vi "Timeout.vi"(11 "Squares type":T1[][](array[typedef])) -> (3 "Clicked Position":i32[](array[numeric]))   [LabVIEW 2019]
uses:
  #typedef_SquareType.ctl
  #typedef_Color.ctl
  #typedef_Piece.ctl
  #typedef_PieceType.ctl
panel:
  out "?":u16[][](array[ring])
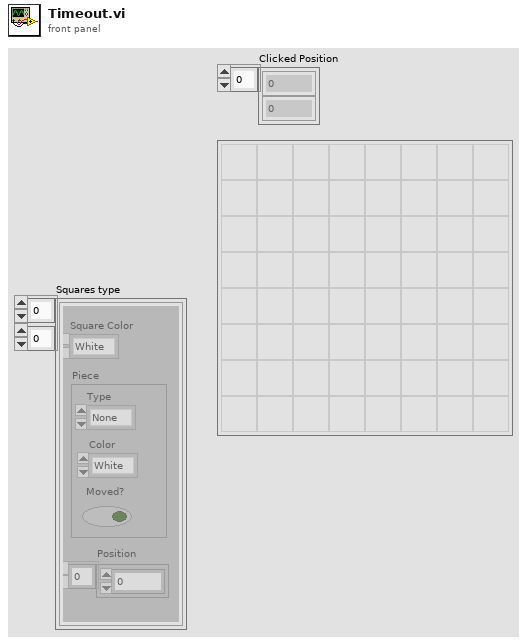
[diagram p1: front panel]
types:
  T1 = typedef "#typedef_SquareType.ctl" = cluster{"Square Color":T2, "Position":i32[], "Piece":T3}
  T2 = typedef "#typedef_Color.ctl" = enum16{"White", "Black"}
  T3 = typedef "#typedef_Piece.ctl" = cluster{"Type":T4, "Color":T2, "Moved?":bool}
  T4 = typedef "#typedef_PieceType.ctl" = enum16{"None", "Pawn", "Knight", "Bishop", "Rook", "Queen", "King"}
  T5 = typedef "LVPositionTypeDef.ctl" = cluster{"Left":i32, "Top":i32}
  T6 = typedef "LVBoundsTypeDef.ctl" = cluster{"Width":u32, "Height":u32}
  T7 = typedef "LVPoint32TypeDef.ctl" = cluster{"Horizontal":i32, "Vertical":i32}
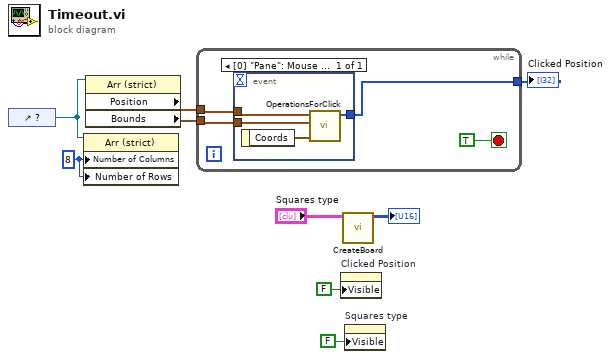
[diagram p0: block diagram]
diagram:
  w4 = u32 8 ("Number of Columns")
  n1 = control-ref of="?"() -> (w1:refnum<vi>)
  n2 = property on="Property Node" class="Arr (strict)"(reference=w1, "Number of Columns"=w4, "Number of Rows"=w4) -> ()  [unwired: 1 in, 2 out]
  n3 = property on="Property Node" class="Arr (strict)"(reference=w1) -> ("Position"=w5:T5, "Bounds"=w6:T6)  [unwired: 1 in, 2 out]
  n4 = while {
    tunnel: w5 -> [w13]
    tunnel: w6 -> [w12]
    tunnel: [w11] -> w7
    stop <- TRUE stop-if-true
    n5 = event shown="[0] \"Pane\": Mouse Down" {
      selector: _ -> [_]
      dyn-events: _ -> [_]
      timeout: _ -> [_]
      tunnel: [w17] -> w11
      tunnel: w13 -> [w14]
      tunnel: w12 -> [w15]
      event Mouse Down {
        n6 = event-data() -> ("Coords"=w16:T7)  [unwired: 1 in]
        n7 = call "OperationsForClick.vi"("Input Coords"=w16, "Input Bounds"=w15, "Input Position"=w14) -> ("Clicked Position"=w17:i32[])  [unwired: 8 in]
      }
    }
  }
  "Clicked Position" <- w7
  n8 = property on="Clicked Position" class="Arr (strict)"("Visible"=FALSE) -> ()  [unwired: 2 in, 2 out]
  n9 = call "CreateBoard.vi"("Squares type"="Squares type") -> ("Board"=→"?":u16[][])  [unwired: 10 in]
  n10 = property on="Squares type" class="Arr (strict)"("Visible"=FALSE) -> ()  [unwired: 2 in, 2 out]
